vi "HF turbidimeter.vi"(4 "State":i16=-1, 5 "Time":dbl format="%.2f", 6 "Sensor Values":dbl[](array[numeric]), 7 "Set Points":dbl[](array[numeric])=[1.0]) -> (0 "required data":T4={"Set Point names"=["data interval (s)", "device ID"], "required number of setpoints"=2, "required number of sensors"=0, "Sensor names"=[]}, 3 "output value":dbl)   [LabVIEW 2019]
uses:
  modbusrtu/ProCoDA MB Request.ctl
  modbusrtu/Read Write.ctl
  modbusrtu/MB ID-Address.ctl
  modbusrtu/MB cmd buffer.ctl
panel:
  in  "MB ID-Address":T1
  in  "ProCoDA MB Read Request":T2 {"Time" format="%.2f"; "# registers" min=1}
  # "Enter the correct information for this control code in the required data structure below. Then make the current value default by right clicking on the border of the data structure. Select \"data operations\" and then select \"make current value default\". These values will be displayed by process controller."
  # "HF turbidimeters have none for parity as default.\nNeed to change to Even!"
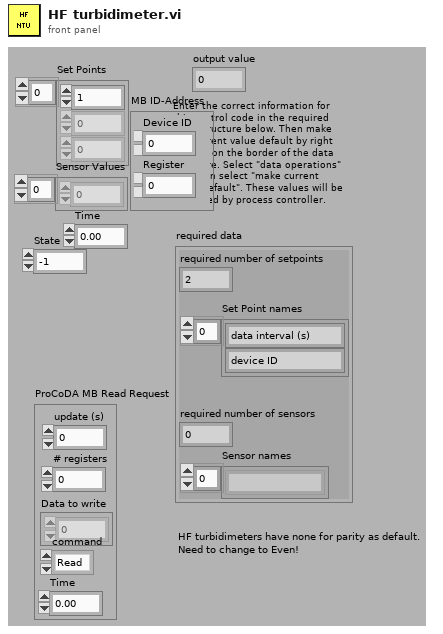
[diagram p1: front panel]
types:
  T1 = typedef "MB ID-Address.ctl" = cluster{"Device ID":u8, "Register":u16}
  T2 = typedef "ProCoDA MB Request.ctl" = cluster{"# registers":u8, "Data to write":u16[], "update (s)":dbl, "command":T3, "Time":dbl}
  T3 = typedef "Read Write.ctl" = enum16{"Read", "Write"}
  T4 = cluster{"Set Point names":string[], "required number of setpoints":u8, "required number of sensors":u8, "Sensor names":string[]}
  T5 = cluster{"Set Points[0]":dbl, "Set Points[1]":dbl}
  T6 = typedef "MB cmd buffer.ctl" = enum16{"ProCoDA", "MB", "MB Next Task", "ProCoDA read 1"}
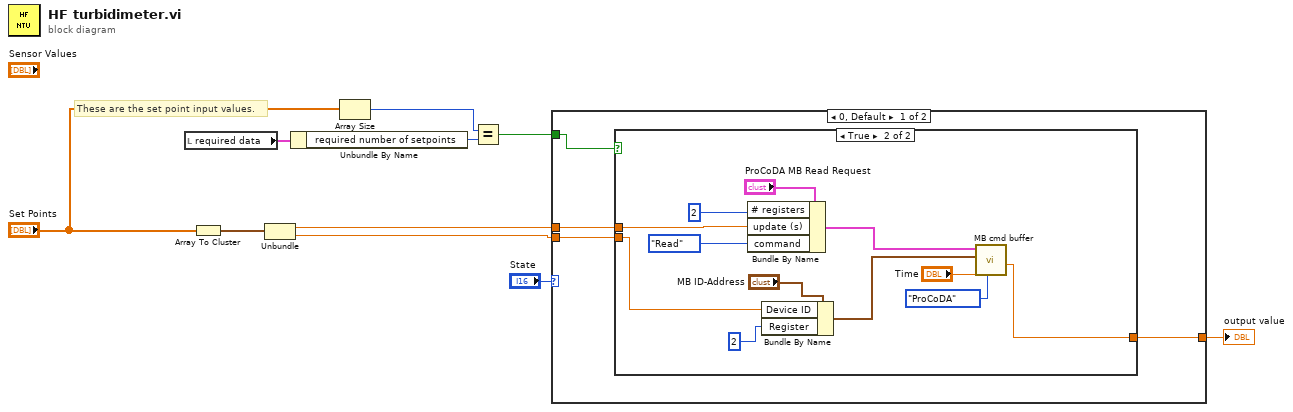
[diagram p0: block diagram]
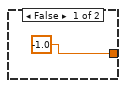
[diagram p2: hidden frame]
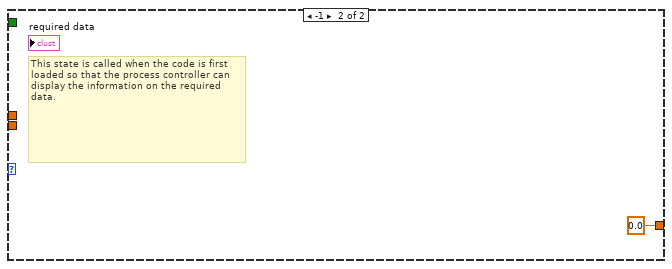
[diagram p3: hidden frame]
diagram:
  # "These are the set point input values."
  n1 = local read "required data"() -> (w6:T4)
  n2 = Array To Cluster(array="Set Points") -> (cluster=w3:T5)
  n3 = Unbundle(w3) -> ("Set Points[0]"=w2:dbl, "Set Points[1]"=w1:dbl)
  n4 = Unbundle By Name(w6) -> ("required number of setpoints"=w5:u8)
  n5 = Array Size(array="Set Points") -> (size(s)=w7:i32)
  n6 = Equal?(x=w7, y=w5) -> (x = y?=w4:bool)
  n7 = case shown="0, Default" "State" {
    tunnel: [w13 0.0 ("fraction on")] -> w9
    tunnel: w4 -> [w14 _]
    tunnel: w2 -> [w12 _]
    tunnel: w1 -> [w11 _]
    frame 0, Default {
      n8 = case shown="True" w14 {
        tunnel: [-1.0 ("fraction on") w18] -> w13
        tunnel: w12 -> [_ w23]
        tunnel: w11 -> [_ w19]
        frame False {
        }
        frame True {
          n9 = Bundle By Name(cluster="ProCoDA MB Read Request", "# registers"=u8 2, "update (s)"=w23, "command"=Read_Write."Read") -> (w25:T2)
          n10 = Bundle By Name(cluster="MB ID-Address", "Device ID"=w19, "Register"=u8 2 ("MB ID-Address.Address")) -> (w16:T1)
          n11 = call "MB cmd buffer.vi"("MB cmd buffer"=MB_cmd_buffer."ProCoDA", "Time"="Time", "MB ID-Address in"=w16, "ProCoDA Request in"=w25) -> ("output value"=w18:dbl)  [unwired: 3 in, 3 out]
        }
      }
    }
    frame -1 {
      # "This state is called when the code is first loaded so that the process controller can display the information on the required data."
    }
  }
  "output value" <- w9
